vi "Read Camera Setup.vi"(8 "error in (no error)":errorcluster, 11 "Hamamatsu_C9100-13 in":refnum<class "Hamamatsu_C9100-13.lvclass">) -> (0 "error out":errorcluster, 2 "Camera Setup":T1={"Analog Gain (0-5)"=4, "Exposure Time"=0.01, "EM Gain (0-255)"=0, "Trigger Polarity"="ATP P", "External Trigger Mode"="EMD E", "Scan Speed"="SSP H", "External Trigger Source"="ESC B", "Scan Mode"="SMD N", "Super Pixel Binning\n(if enabled in Scan Mode)"="SPX 1", "Camera Sub-array acquisition region\n(if enabled in scan mode)"={"Left"=0, "Top"=0, "Width"=0, "Height"=0}, "Use camera?"=FALSE, "# image buffers"=100, "shots per measurement"=100, "Force images to U16"=FALSE, "Low Light Sensitivity"="LLS 0", "cooling"="CSW F", "fan"="FAN F", "Frame Grabber acquisition region"={"Left"=0, "Top"=0, "Right"=0, "Bottom"=0}} {"Frame Grabber acquisition region"."Bottom" max=512 step=1; "Frame Grabber acquisition region"."Right" max=512 step=1; "Frame Grabber acquisition region"."Top" max=512 step=1; "Frame Grabber acquisition region"."Left" max=512 step=1; "shots per measurement" min=0 step=1; "# image buffers" min=0 step=1; "Camera Sub-array acquisition region\n(if enabled in scan mode)"."Height" min=16 max=512 step=16; "Camera Sub-array acquisition region\n(if enabled in scan mode)"."Width" min=16 max=512 step=16; "Camera Sub-array acquisition region\n(if enabled in scan mode)"."Top" max=496 step=16; "Camera Sub-array acquisition region\n(if enabled in scan mode)"."Left" max=496 step=16; "Analog Gain (0-5)" max=5 step=1}, 3 "Hamamatsu_C9100-13 out":refnum<class "Hamamatsu_C9100-13.lvclass">)   [LabVIEW 2013, in "Hamamatsu_C9100-13.lvclass"]
uses:
  Hamamatsu_C9100-13.lvclass
  camera_setup.ctl
  Hamamatsu_C9100-13.lvclass/Hamamatsu_C9100-13.ctl
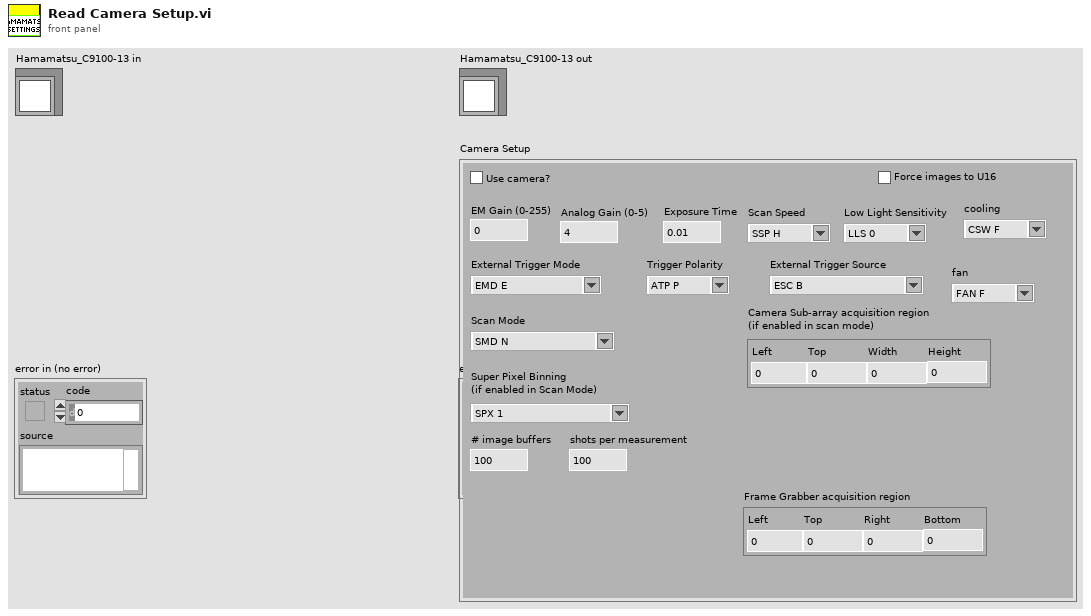
[diagram p1: front panel]
types:
  T1 = typedef "Hamamatsu_C9100-13.lvclass/camera_setup.ctl" = cluster{"Analog Gain (0-5)":u8, "Exposure Time":dbl, "EM Gain (0-255)":u8, "Trigger Polarity":string, "External Trigger Mode":string, "Scan Speed":string, "External Trigger Source":string, "Scan Mode":string, "Super Pixel Binning\n(if enabled in Scan Mode)":string, "Camera Sub-array acquisition region\n(if enabled in scan mode)":cluster{"Left":u16, "Top":u16, "Width":u16, "Height":u16}, "Use camera?":bool, "# image buffers":i32, "shots per measurement":i32, "Force images to U16":bool, "Low Light Sensitivity":string, "cooling":string, "fan":string, "Frame Grabber acquisition region":cluster{"Left":i32, "Top":i32, "Right":i32, "Bottom":i32}}
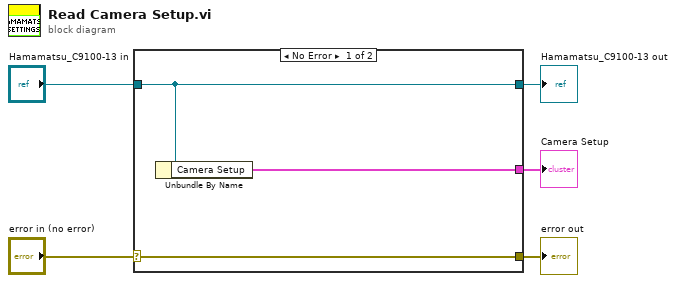
[diagram p0: block diagram]
diagram:
  n1 = case shown="No Error" "error in (no error)" {
    selector: "error in (no error)" -> [w8 w9]
    tunnel: [w8 w9] -> w4
    tunnel: [w7 w10] -> w2
    tunnel: "Hamamatsu_C9100-13 in" -> [w7 w10]
    tunnel: [w6 _] -> w1
    frame No Error {
      n2 = Unbundle By Name(w7) -> ("Camera Setup"=w6:T1)
    }
    frame Error {
    }
  }
  "error out" <- w4
  "Hamamatsu_C9100-13 out" <- w2
  "Camera Setup" <- w1
